vi "Geometric PF.vi"(10 "p":dbl=0.5, 11 "x":i32=1) -> (0 "error":i32, 3 "prob(x)":dbl=0.25)   [LabVIEW 2014, in "NI_Gmath.lvlib"]
doc: "Computes the discrete probability function (PF), or the probability that the random variate X, where X describes the selected distribution type, takes on the value <B>n</B>. You must manually select the polymorphic instance to use."
uses:
  NI_Gmath.lvlib
panel:
  # "Geometric PF"
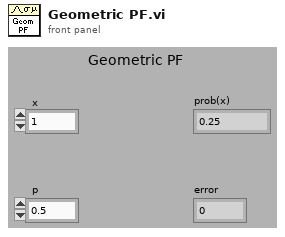
[diagram p1: front panel]
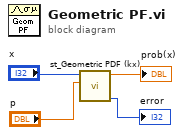
[diagram p0: block diagram]
diagram:
  n1 = call "st_Geometric PDF (kx).vi"("p"="p", "x"="x") -> ("error"=→"error":i32, "pdf(x)"=→"prob(x)":dbl)  [unwired: 8 in]
